vi "stop_sweep.vi"(8 "error in (no error)":errorcluster, 11 "ScanModeDL091001Scaffold in":refnum<class "ImagingModeDL091001Scaffold.lvclass">) -> (0 "error out":errorcluster, 3 "ScanModeDL091001Scaffold out":refnum<class "ImagingModeDL091001Scaffold.lvclass">)   [LabVIEW 2010, in "ImagingModeDL091001Scaffold.lvclass"]
uses:
  ImagingModeDL091001Scaffold.lvclass
  ImagingModeDL090923Scaffold/ImagingModeDL090923Scaffold/ImagingModeDL090923Scaffold.lvclass
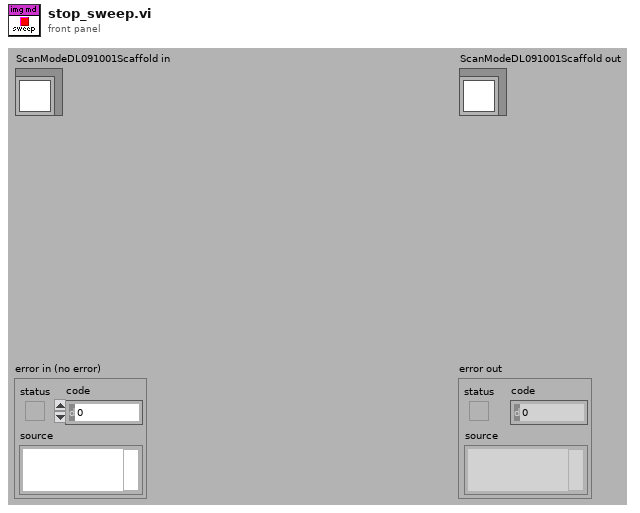
[diagram p1: front panel]
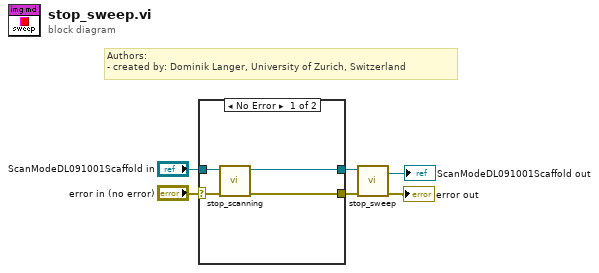
[diagram p0: block diagram]
diagram:
  # "Authors: \n- created by: Dominik Langer, University of Zurich, Switzerland"
  n1 = case shown="No Error" "error in (no error)" {
    selector: "error in (no error)" -> [w10 w12]
    tunnel: [w8 w12] -> w3
    tunnel: [w7 w11] -> w1
    tunnel: "ScanModeDL091001Scaffold in" -> [w9 w11]
    frame No Error {
      n2 = call-dynamic "stop_scanning.vi"("error in (no error)"=w10, "ScanModeDL090923Scaffold in"=w9) -> ("error out"=w8:errorcluster, "ScanModeDL090923Scaffold out"=w7:refnum<class "ImagingModeDL091001Scaffold.lvclass">)  [unwired: 8 in]
    }
    frame Error {
    }
  }
  n3 = call-parent "stop_sweep.vi"("error in (no error)"=w3, "ScanModeDL090923Scaffold in"=w1) -> ("error out"=→"error out":errorcluster, "ScanModeDL090923Scaffold out"=→"ScanModeDL091001Scaffold out":refnum<class "ImagingModeDL091001Scaffold.lvclass">)  [unwired: 8 in]
